vi "DAQ_AO_WF.vi"(0 "Exposure time (s)":dbl=0.1, 5 "Readout time (s)":dbl=0.1, 7 "A01_voltage":dbl=1.0, 9 "A02_voltage":dbl=1.0, 11 "error in":errorcluster caption="entrée d'erreur") -> (4 "AO WF":waveform(dbl)[](graph), 6 "Dimension":i32, 15 "error out":errorcluster caption="sortie d'erreur")   [LabVIEW 2025]
uses:
  Controls/TypeDef_FGV.ctl
panel:
  out "tableau ajouté":waveform(dbl)[](array[waveform])
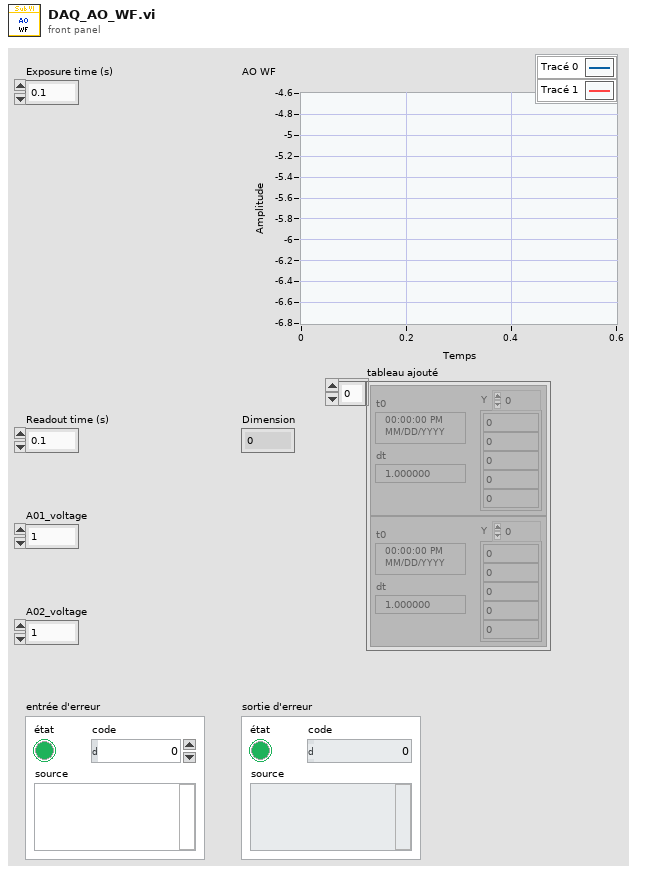
[diagram p1: front panel]
types:
  T1 = typedef "TypeDef_FGV.ctl" = enum16{"Initialize", "Write", "Read"}
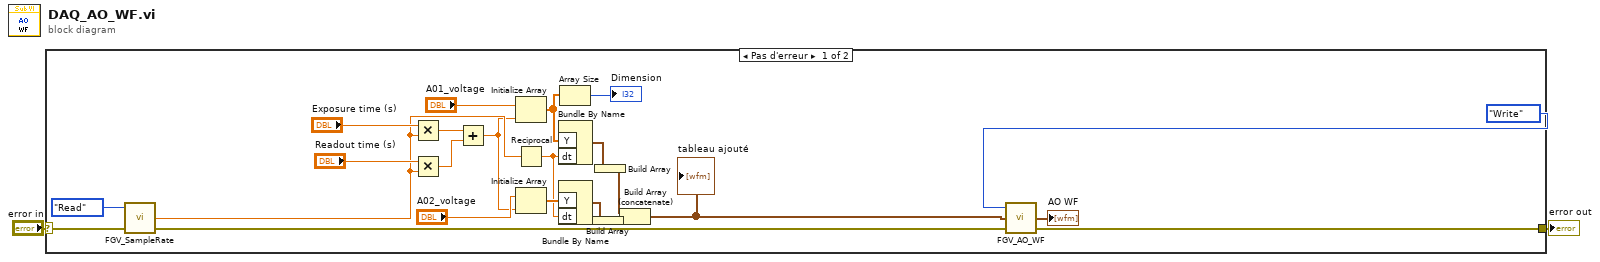
[diagram p0: block diagram]
diagram:
  n1 = case shown="Pas d'erreur" "error in" {
    selector: "error in" -> [w25 w26]
    tunnel: [w18 w26] -> w1
    frame No Error {
      n2 = call "FGV_SampleRate.vi"("error in"=w25, "Action"=TypeDef_FGV."Read") -> ("error out"=w15:errorcluster, "CO task"=w20:dbl)  [unwired: 2 in]
      n3 = Multiply(x="Exposure time (s)", y=w20) -> (x*y=w17:dbl)
      n4 = Multiply(x="Readout time (s)", y=w20) -> (x*y=w16:dbl)
      n5 = Add(x=w17, y=w16) -> (x+y=w12:dbl)
      n6 = Initialize Array("A01_voltage", w12) -> (w11:dbl[])
      n7 = Reciprocal(x=w20) -> (1/x=w9:dbl)
      n8 = Initialize Array("A02_voltage", w12) -> (w10:dbl[])
      n9 = Bundle By Name("Y"=w11, "dt"=w9) -> (w8:waveform(dbl))  [unwired: 1 in]
      n10 = Bundle By Name("Y"=w10, "dt"=w9) -> (w7:waveform(dbl))  [unwired: 1 in]
      n11 = Array Size(array=w11) -> (size(s)=→"Dimension":i32)
      n12 = Build Array(w7) -> (w3:waveform(dbl)[])
      n13 = Build Array(w8) -> (w4:waveform(dbl)[])
      n14 = Build Array (concatenate)(w4, w3) -> (w6:waveform(dbl)[])
      "tableau ajouté" <- w6
      n15 = call "FGV_AO_WF.vi"("error in 2"=w15, "AO WF 3"=w6, "Action 2"=TypeDef_FGV."Write" ("Action")) -> ("error out 2"=w18:errorcluster, "AO WF 2"=→"AO WF":waveform(dbl)[])  [unwired: 1 in]
    }
    frame Error {
    }
  }
  "error out" <- w1
